vi "_Cluster AutoSizing Dialog.vi"() -> (0 "cancelled?":bool=TRUE, 1 "Recursively (dup)":bool, 3 "type":T1(ring))   [LabVIEW 2017, in "Cluster AutoSizing.lvlib"]
uses:
  Cluster AutoSizing.lvlib
panel:
  in  "Recursively":bool
  in  "Arrange Veritcally":bool
  in  "Arrange Horizontally":bool
  in  "Size to fit":bool
  in  "None":bool
  # "1"
  # "2"
  # "3"
  # "4"
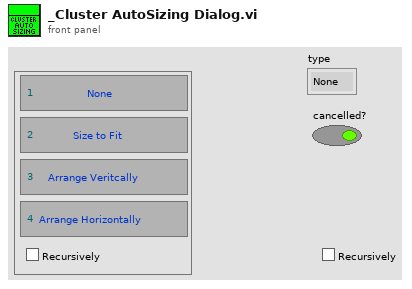
[diagram p1: front panel]
types:
  T1 = enum16{"None", "Size to Fit", "Arrange Horizontally", "Arrange Veritcally"}
  T2 = typedef "eventvkey.ctl" = enum16{"ASCII", "Enter", "Return", "Shift", "Ctrl", "Alt", "Cmd", "Opt", "Caps", "NumLock", "Clear", "Break", "Up", "Down", "Left", "Right", "Insert", "Delete", "Home", "End", "PageUp", "PageDown", "Escape", "Help", "Pause", "ScrollLock", "F1", "F2", "F3", "F4", "F5", "F6", "F7", "F8", "F9", "F10", "F11", "F12", "F13", "F14", "F15", "F16", "F17", "F18", "F19", "F20", "F21", "F22", "F23", "F24", "Play", "VolumeUp", "VolumeDown", "Mute", "Two Byte Char"}
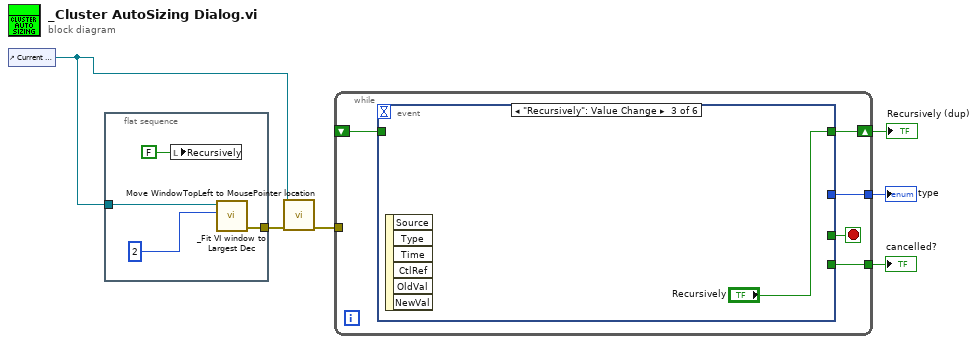
[diagram p0: block diagram]
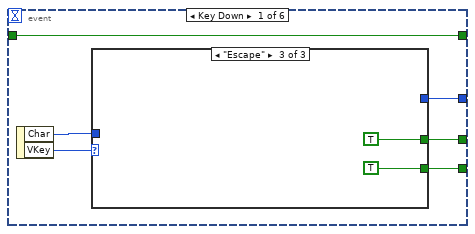
[diagram p2: hidden frame]
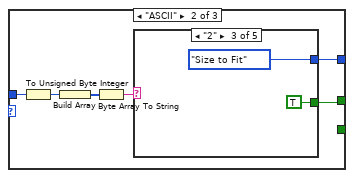
[diagram p4: hidden frame]
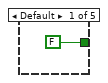
[diagram p5: hidden frame]
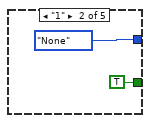
[diagram p6: hidden frame]
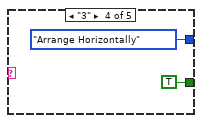
[diagram p7: hidden frame]
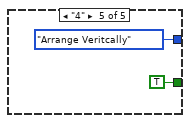
[diagram p8: hidden frame]
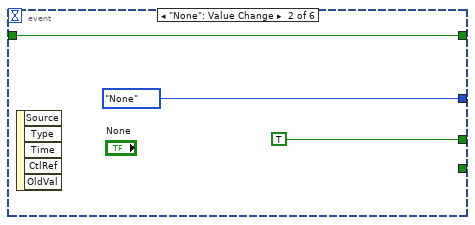
[diagram p9: hidden frame]
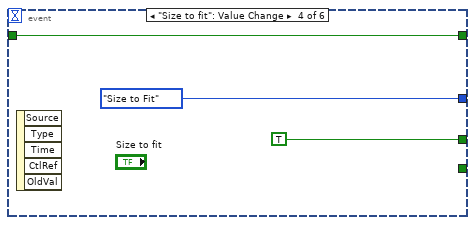
[diagram p10: hidden frame]
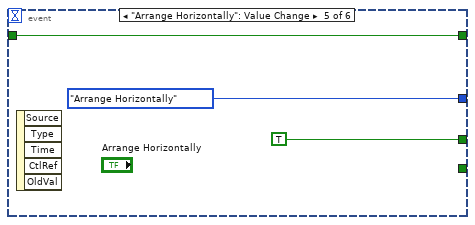
[diagram p11: hidden frame]
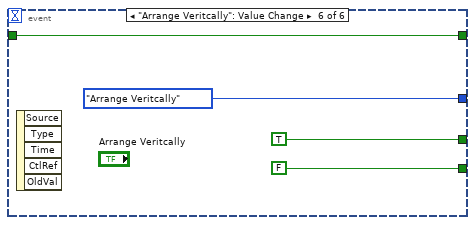
[diagram p12: hidden frame]
diagram:
  n1 = control-ref of="Current VI Reference"() -> (w1:refnum<vi>)
  n2 = flat-sequence {
    tunnel: [w9] -> w2
    tunnel: w1 -> [w7]
    frame #0 {
      n3 = local write "Recursively"(FALSE ("Recursively")) -> ()
      n4 = call "_Fit VI window to Largest Dec.vi"("border spacing (2 px)"=2, "VI Ref (calling VI)"=w7) -> ("error out"=w9:errorcluster)  [unwired: 4 in, 1 out]
    }
  }
  n5 = call "Move WindowTopLeft to MousePointer location.vi"("error in (no error)"=w2, "VIRef"=w1) -> ("error out"=w3:errorcluster)  [unwired: 9 in]
  n6 = while {
    tunnel: [w14] -> w5
    tunnel: [w13] -> w6
    shift-right: [w12] -> w4
    shift-left: _ -> [w11]
    tunnel: w3 -> [_]
    stop <- w15 stop-if-true
    n7 = event shown="[2] \"Recursively\": Value Change" {
      selector: _ -> [_ _ _ _ _ _]
      dyn-events: _ -> [_ _ _ _ _ _]
      timeout: _ -> [_ _ _ _ _ _]
      tunnel: [w20 TRUE _ TRUE TRUE TRUE] -> w15
      tunnel: [w19 _ _ _ _ FALSE] -> w14
      tunnel: [w17 T1."None" _ T1."Size to Fit" T1."Arrange Horizontally" T1."Arrange Veritcally"] -> w13
      tunnel: [w16 w39 "Recursively" w43 w46 w49] -> w12
      tunnel: w11 -> [w16 w39 _ w43 w46 w49]
      event Key Down {
        n8 = event-data() -> ("Char"=w18:i16, "VKey"=w21:T2)  [unwired: 1 in]
        n9 = case shown="\"Escape\"" w21 {
          tunnel: [_ w22 TRUE] -> w20
          tunnel: [_ _ TRUE] -> w19
          tunnel: w18 -> [_ w25 _]
          tunnel: [_ w23 _] -> w17
          frame Default {
          }
          frame "ASCII" {
            n10 = To Unsigned Byte Integer(number=w25) -> (unsigned 8bit integer=w26:u8)
            n11 = Build Array(w26) -> (w27:u8[])
            n12 = Byte Array To String(unsigned byte array=w27) -> (string=w24:string)
            n13 = case shown="\"2\"" w24 {
              tunnel: [_ T1."None" T1."Size to Fit" T1."Arrange Horizontally" T1."Arrange Veritcally"] -> w23
              tunnel: [FALSE TRUE TRUE TRUE TRUE] -> w22
              frame Default {
              }
              frame "1" {
              }
              frame "2" {
              }
              frame "3" {
              }
              frame "4" {
              }
            }
          }
          frame "Escape" {
          }
        }
      }
      event "None": Value Change {
        n14 = event-data() -> ()  [unwired: 1 in, 5 out]
      }
      event "Recursively": Value Change {
        n15 = event-data() -> ()  [unwired: 1 in, 6 out]
      }
      event "Size to fit": Value Change {
        n16 = event-data() -> ()  [unwired: 1 in, 5 out]
      }
      event "Arrange Horizontally": Value Change {
        n17 = event-data() -> ()  [unwired: 1 in, 5 out]
      }
      event "Arrange Veritcally": Value Change {
        n18 = event-data() -> ()  [unwired: 1 in, 5 out]
      }
    }
  }
  "type" <- w6
  "cancelled?" <- w5
  "Recursively (dup)" <- w4
